vi "Get State.vi"(8 "error in (no error)":errorcluster, 11 "Pulse Controller in":refnum<class "Instrument Actor.lvclass">) -> (0 "error out":errorcluster, 1 "Result ready":bool, 2 "Armed":bool, 3 "Pulse Controller out":refnum<class "Instrument Actor.lvclass">)   [LabVIEW 2016, in "Instrument Actor.lvclass"]
uses:
  Instrument Actor.lvclass
  Instrument Actor.lvclass/Instrument Actor.ctl
  Read Instrument driver.vi
  Write Instrument driver.vi
  NHMFL_Core/Libraries/Instruments/Instrument Driver/Instrument Driver.lvclass
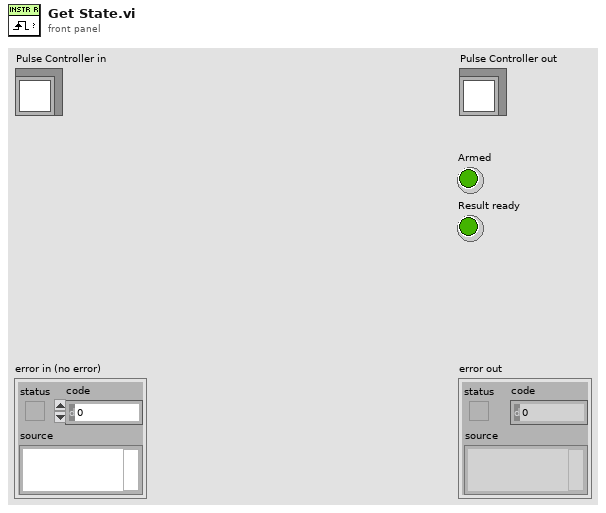
[diagram p1: front panel]
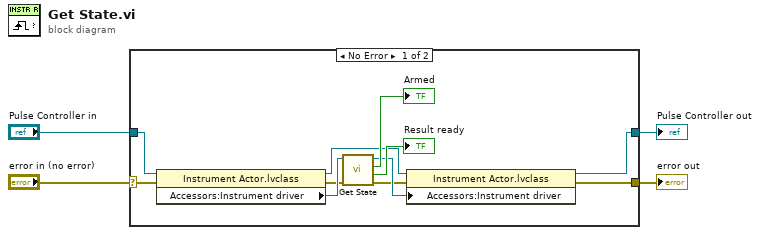
[diagram p0: block diagram]
diagram:
  n1 = case shown="No Error" "error in (no error)" {
    selector: "error in (no error)" -> [w11 w17]
    tunnel: [w6 w17] -> w3
    tunnel: [w5 w16] -> w1
    tunnel: "Pulse Controller in" -> [w14 w16]
    frame No Error {
      n2 = property class="Instrument Actor.lvclass"(reference=w14, error in=w11) -> (reference out=w9:refnum<class "Instrument Actor.lvclass">, error out=w10:errorcluster, "Accessors:Instrument driver"=w12:refnum<class "Instrument Driver.lvclass">)
      n3 = call-dynamic "Get State.vi"("error in (no error)"=w10, "Instrument Driver in"=w12) -> ("error out"=w7:errorcluster, "Data ready"=→"Result ready":bool, "Armed"=→"Armed":bool, "Instrument Driver out"=w8:refnum<class "Instrument Driver.lvclass">)  [unwired: 4 in, 2 out]
      n4 = property class="Instrument Actor.lvclass"(reference=w9, error in=w7, "Accessors:Instrument driver"=w8) -> (reference out=w5:refnum<class "Instrument Actor.lvclass">, error out=w6:errorcluster)
    }
    frame Error {
    }
  }
  "error out" <- w3
  "Pulse Controller out" <- w1
